vi "SV Get By Measurement Type (tach) (N Ch).vi"(0 "scaled signals [EU]":waveform(dbl)[](array[waveform])) -> (4 "scaled signals with tachometer channels deleted":waveform(dbl)[](array[waveform]), 6 "number of tachometer channels":i32, 8 "tachometer channels":waveform(dbl)[](array[waveform]))   [LabVIEW 2017]
uses:
  <vilib>/addons/_NISVFA/_Shared subVIs/Controls/SV Channel Properties.ctl
panel:
  out "maximum order":i32[](array[numeric])
  out "threshold":dbl[](array[numeric])
  out "rotation direction":u16[](array[ring]) items=["CCW", "CW"]
  out "pulses per rev":i32[](array[numeric])
  out "slope":u16[](array[ring]) items=["Rising", "Falling"]
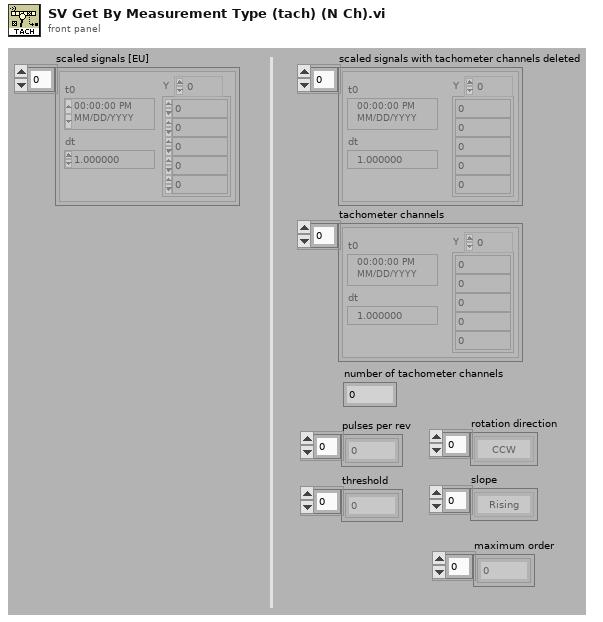
[diagram p1: front panel]
types:
  T1 = typedef "SV Channel Properties.ctl" = u16
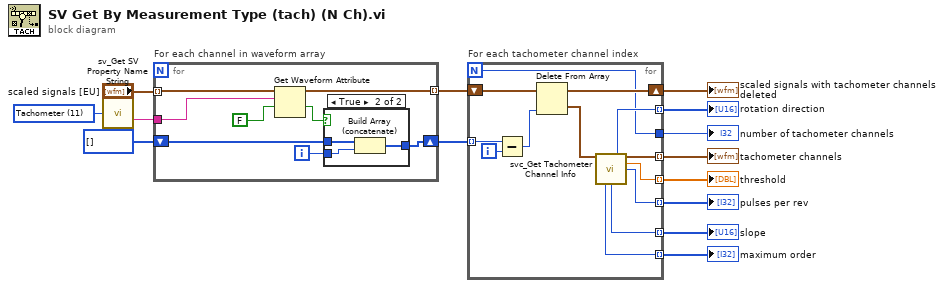
[diagram p0: block diagram]
diagram:
  w5 = T1 11 items=["Engineering units", "Custom unit label", "Weighting filter", "Pregain", "Octave standard", "Octave bandwidth", "Octave low band", "Octave high band", "Spectrum skewed", "Samples / revolution", "Order", "Tachometer", "Pulses Per Revolution", "Rotation Direction", "Probe Angle", "Pair", "Channel Alias"] ("property")
  n1 = call <vilib>:"sv_Get SV Property Name String.vi"("property"=w5) -> ("WDT attribute name"=w4:string)  [unwired: 13 in, 1 out]
  n2 = for "For each channel in waveform array" {
    tunnel: "scaled signals [EU]" -> [w22] mode=indexing
    shift-right: [w18] -> w12
    shift-left: i32[] [] -> [w20]
    tunnel: w4 -> [w16]
    tunnel: [w15] -> w2 mode=indexing
    i -> [w19]
    n3 = Get Waveform Attribute(5:FALSE, 6:w16, 7:w22) -> (1:w21:bool, 3:w15:waveform(dbl))  [unwired: 1 in, 2 out]
    n4 = case shown="True" w21 {
      tunnel: w20 -> [w23 w26]
      tunnel: w19 -> [_ w25]
      tunnel: [w23 w24] -> w18
      frame False {
      }
      frame True {
        n5 = Build Array (concatenate)(w26, w25) -> (w24:i32[])
      }
    }
  }
  n6 = for "For each tachometer channel index" {
    N -> [w27]
    shift-right: [w38] -> w13
    shift-left: w2 -> [w39]
    tunnel: w12 -> [w37] mode=indexing
    tunnel: [w31] -> w10 mode=indexing
    tunnel: [w30] -> w9 mode=indexing
    tunnel: [w33] -> w8 mode=indexing
    tunnel: [w29] -> w11 mode=indexing
    tunnel: [w32] -> w6 mode=indexing
    tunnel: [w28] -> w7 mode=indexing
    tunnel: [w27] -> w1
    i -> [w35]
    n7 = Subtract(x=w37, y=w35) -> (x-y=w36:i32)
    n8 = Delete From Array(array=w39, index=w36) -> (deleted portion=w34:waveform(dbl), array with subset deleted=w38:waveform(dbl)[])  [unwired: 1 in]
    n9 = call <vilib>:"svc_Get Tachometer Channel Info.vi"("Tachometer Channel in"=w34) -> ("rotation direction"=w30:u16, "Tachometer Channel out"=w28:waveform(dbl), "Threshold"=w33:dbl, "Pulses Per Rev"=w31:i32, "Max Order"=w32:i32, "Slope"=w29:u16)  [unwired: 9 in]
  }
  "scaled signals with tachometer channels deleted" <- w13
  "tachometer channels" <- w7
  "number of tachometer channels" <- w1
  "slope" <- w11
  "pulses per rev" <- w10
  "rotation direction" <- w9
  "threshold" <- w8
  "maximum order" <- w6
